vi "logicBox.vi"(9 "Arg":dbl, 10 "Mod":dbl, 11 "TrackState":bool) -> (1 "Arg":dbl, 2 "Mod":dbl, 3 "State":enum16{"notTracked", "NullMessage", "OK"}(ring))   [LabVIEW 2012]
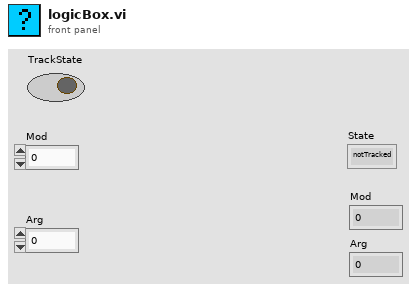
[diagram p1: front panel]
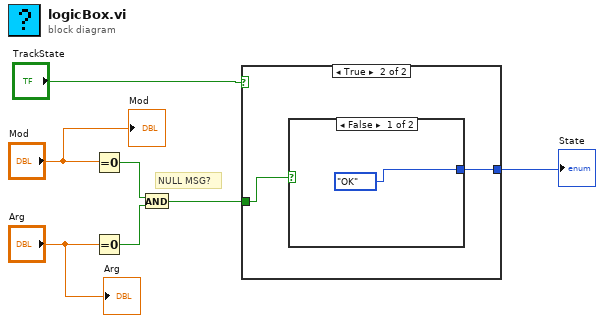
[diagram p0: block diagram]
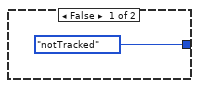
[diagram p2: hidden frame]
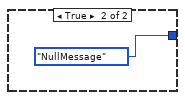
[diagram p3: hidden frame]
diagram:
  # "NULL MSG?"
  n1 = Equal To 0?(x="Mod") -> (x = 0?=w7:bool)
  n2 = Equal To 0?(x="Arg") -> (x = 0?=w6:bool)
  n3 = And(x=w7, y=w6) -> (x .and. y?=w4:bool)
  n4 = case shown="True" "TrackState" {
    tunnel: [enum16{"notTracked", "NullMessage", "OK"}."notTracked" w9] -> w3
    tunnel: w4 -> [_ w10]
    frame False {
    }
    frame True {
      n5 = case shown="False" w10 {
        tunnel: [enum16{"notTracked", "NullMessage", "OK"}."OK" enum16{"notTracked", "NullMessage", "OK"}."NullMessage"] -> w9
        frame False {
        }
        frame True {
        }
      }
    }
  }
  "State" <- w3
  "Arg" <- "Arg"
  "Mod" <- "Mod"
